vi "Cmd_U16U32U16U32.vi"(4 "Arg3":i16, 5 "Arg2":u32 max=127 step=1, 6 "Arg4":u32, 7 "Arg1":u16 max=127 step=1, 8 "error in (no error)":errorcluster, 9 "Cmd":u8, 10 "Address":u8, 11 "VISA Refnum in":refnum<visa-resource-name>) -> (0 "error out":errorcluster, 2 "Valid":bool, 3 "VISA Refnum out":refnum<visa-resource-name>)   [LabVIEW 2015, in "Ion Motion Roboclaw.lvlib"]
uses:
  <instrlib>/Ion Motion Roboclaw/Ion Motion Roboclaw.lvlib
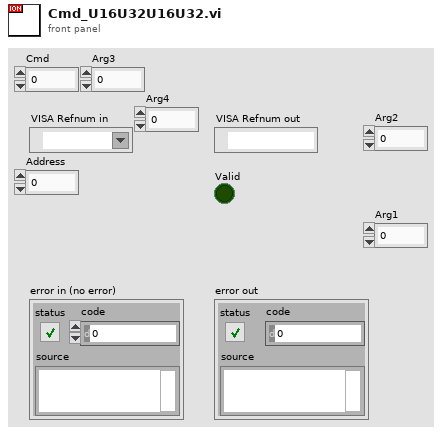
[diagram p1: front panel]
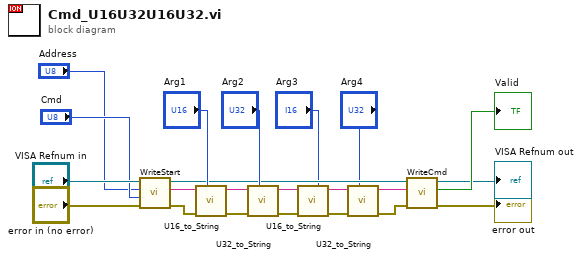
[diagram p0: block diagram]
diagram:
  n1 = call <instrlib>:"WriteStart.vi"("error in (no error)"="error in (no error)", "Cmd"="Cmd", "Address"="Address", "VISA Refnum in"="VISA Refnum in") -> ("error out"=w15:errorcluster, "String Out"=w16:string, "VISA Refnum out"=w9:refnum<visa-resource-name>)  [unwired: 5 in]
  n2 = call <instrlib>:"U16_to_String.vi"("number"="Arg1", "error in (no error)"=w15, "String In"=w16) -> ("error out"=w14:errorcluster, "String Out"=w13:string)  [unwired: 5 in]
  n3 = call <instrlib>:"U32_to_String.vi"("number"="Arg2", "error in (no error)"=w14, "String In"=w13) -> ("error out"=w8:errorcluster, "String Out"=w3:string)  [unwired: 5 in]
  n4 = call <instrlib>:"U16_to_String.vi"("number"="Arg3", "error in (no error)"=w8, "String In"=w3) -> ("error out"=w7:errorcluster, "String Out"=w4:string)  [unwired: 5 in]
  n5 = call <instrlib>:"U32_to_String.vi"("number"="Arg4", "error in (no error)"=w7, "String In"=w4) -> ("error out"=w6:errorcluster, "String Out"=w5:string)  [unwired: 5 in]
  n6 = call <instrlib>:"WriteCmd.vi"("error in (no error)"=w6, "write buffer"=w5, "VISA Refnum in"=w9) -> ("error out"=→"error out":errorcluster, "Valid"=→"Valid":bool, "VISA Refnum out"=→"VISA Refnum out":refnum<visa-resource-name>)  [unwired: 2 in]
